vi "Read Serial Session.vi"(8 "error in (no error)":errorcluster, 11 "PPT in":refnum<class "PPT.lvclass">) -> (0 "error out":errorcluster, 2 "Session Handle":T1, 3 "PPT out":refnum<class "PPT.lvclass">)   [LabVIEW 2015, in "PPT Library.lvlib" / "PPT.lvclass"]
uses:
  PPT.lvclass
  <vilib>/MSR Consulting, LLC/ESF/Typedefs/Session Handle.ctl
  <vilib>/MSR Consulting, LLC/ESF/Session - Root.lvclass
  PPT.lvclass/PPT.ctl
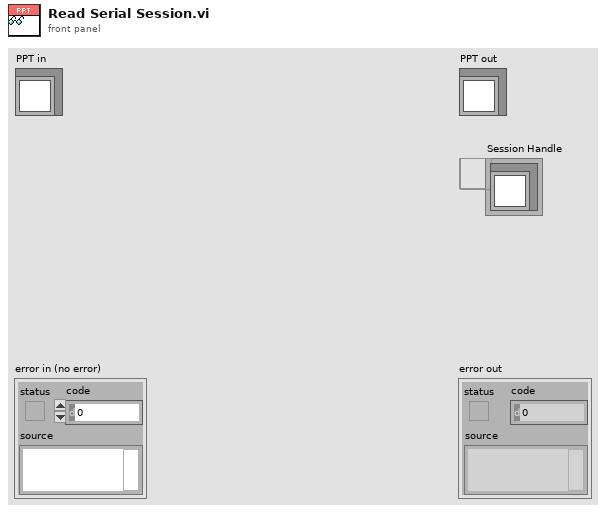
[diagram p1: front panel]
types:
  T1 = typedef "Session - Root.lvclass/Session Handle.ctl" = refnum<data-value>
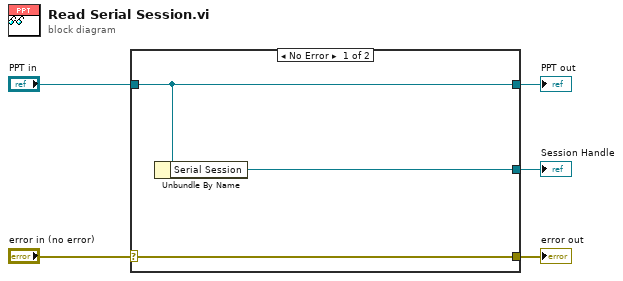
[diagram p0: block diagram]
diagram:
  n1 = case shown="No Error" "error in (no error)" {
    selector: "error in (no error)" -> [w8 w9]
    tunnel: [w8 w9] -> w4
    tunnel: [w7 w10] -> w2
    tunnel: "PPT in" -> [w7 w10]
    tunnel: [w6 _] -> w1
    frame No Error {
      n2 = Unbundle By Name(w7) -> ("Serial Session"=w6:T1)
    }
    frame Error {
    }
  }
  "error out" <- w4
  "PPT out" <- w2
  "Session Handle" <- w1
